vi "Run TCS.vi"(8 "error in (no error)":errorcluster, 11 "SPARC4_GEI in":refnum<class "SPARC4_GEI.lvclass">) -> (0 "error out":errorcluster, 3 "SPARC4_GEI out":refnum<class "SPARC4_GEI.lvclass">)   [LabVIEW 2018, in "SPARC4_GEI.lvclass"]
uses:
  SPARC4_GEI.lvclass
  SPARC4_GEI.lvclass/SPARC4_GEI.ctl
  Filter_Wheel/Filter_Wheel.lvclass/Filter_Wheel.ctl
  State Machine/State Machine.lvclass
  TCS/TCS.lvclass
  Channel GUI/Channel GEI.lvclass
  Filter_Wheel/Filter_Wheel.lvclass
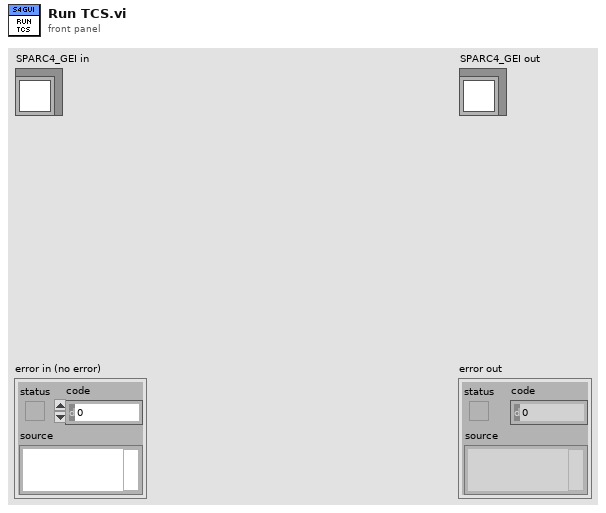
[diagram p1: front panel]
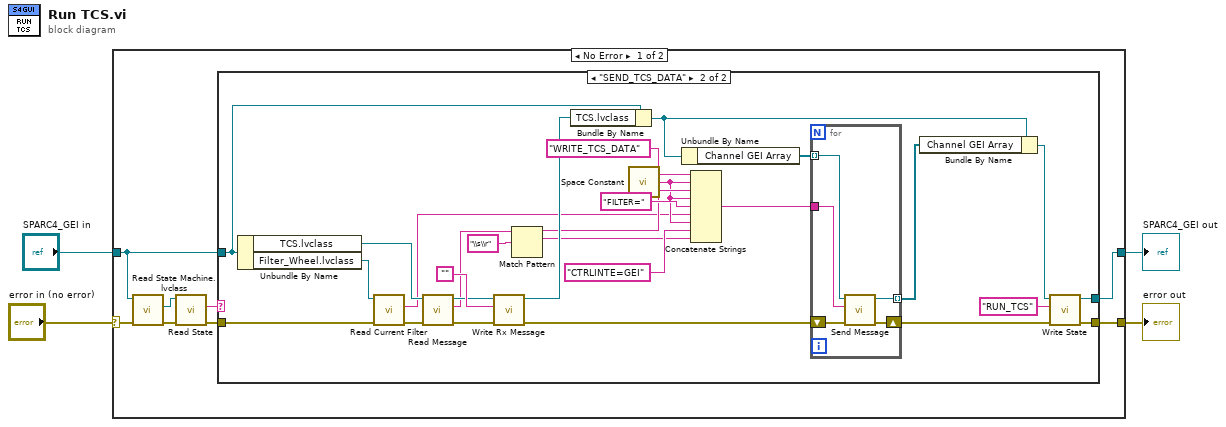
[diagram p0: block diagram]
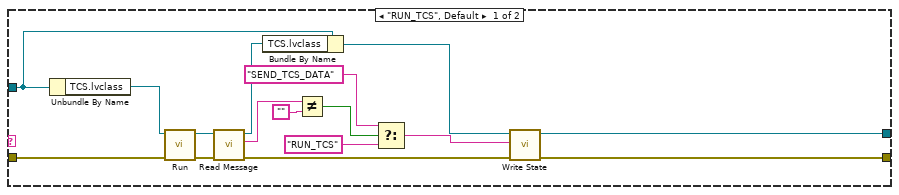
[diagram p2: hidden frame]
diagram:
  n1 = case shown="No Error" "error in (no error)" {
    selector: "error in (no error)" -> [w8 w63]
    tunnel: [w11 w63] -> w3
    tunnel: [w12 w62] -> w2
    tunnel: "SPARC4_GEI in" -> [w5 w62]
    frame No Error {
      n2 = call "Read State Machine.lvclass.vi"("error in (no error)"=w8, "SPARC4_GUI in"=w5) -> ("error out"=w9:errorcluster, "State Machine.lvclass"=w10:refnum<class "State Machine.lvclass">)  [unwired: 7 in, 1 out]
      n3 = call-dynamic "Read State.vi"("error in (no error)"=w9, "State Machine in"=w10) -> ("error out"=w7:errorcluster, "State"=w6:string)  [unwired: 7 in, 1 out]
      n4 = case shown="\"SEND_TCS_DATA\"" w6 {
        tunnel: [w28 w51] -> w12
        tunnel: [w27 w50] -> w11
        tunnel: w7 -> [w15 w31]
        tunnel: w5 -> [w13 w41]
        frame "RUN_TCS", Default {
          n5 = Unbundle By Name(w13) -> ("TCS.lvclass"=w16:refnum<class "TCS.lvclass">)
          n6 = call "Run.vi"("error in (no error)"=w15, "TCS in"=w16) -> ("error out"=w25:errorcluster, "TCS out"=w26:refnum<class "TCS.lvclass">)  [unwired: 8 in]
          n7 = call "Read Message.vi"("error in (no error)"=w25, "TCS in"=w26) -> ("error out"=w23:errorcluster, "Rx Message"=w18:string, "TCS out"=w24:refnum<class "TCS.lvclass">)  [unwired: 7 in]
          n8 = Bundle By Name(cluster=w13, "TCS.lvclass"=w24) -> (w14:refnum<class "SPARC4_GEI.lvclass">)
          n9 = Not Equal?(x=w18, y="") -> (x != y?=w19:bool)
          n10 = Select(t="SEND_TCS_DATA", s=w19, f="RUN_TCS") -> (s? t:f=w22:string)
          n11 = call "Write State.vi"("error in (no error)"=w23, "State"=w22, "SPARC4_GEI in"=w14) -> ("error out"=w27:errorcluster, "SPARC4_GEI out"=w28:refnum<class "SPARC4_GEI.lvclass">)  [unwired: 7 in]
        }
        frame "SEND_TCS_DATA" {
          n12 = Unbundle By Name(w41) -> ("TCS.lvclass"=w42:refnum<class "TCS.lvclass">, "Filter_Wheel.lvclass"=w32:refnum<class "Filter_Wheel.lvclass">)
          n13 = call "Read Current Filter.vi"("error in (no error)"=w31, "Filter_Wheel in"=w32) -> ("error out"=w30:errorcluster, "Current Filter"=w29:string)  [unwired: 7 in, 1 out]
          n14 = call "Read Message.vi"("error in (no error)"=w30, "TCS in"=w42) -> ("error out"=w47:errorcluster, "Rx Message"=w38:string, "TCS out"=w48:refnum<class "TCS.lvclass">)  [unwired: 7 in]
          n15 = call "Write Rx Message.vi"("error in (no error)"=w47, "Rx Message"="", "TCS in"=w48) -> ("error out"=w54:errorcluster, "TCS out"=w53:refnum<class "TCS.lvclass">)  [unwired: 7 in]
          n16 = Match Pattern(string=w38, regular expression="\\s\\r") -> (before substring=w36:string, match substring=w33:string)  [unwired: 1 in, 2 out]
          n17 = Bundle By Name(cluster=w41, "TCS.lvclass"=w53) -> (w55:refnum<class "SPARC4_GEI.lvclass">)
          n18 = call <vilib>:"Space Constant.vi"() -> ("String"=w35:string)
          n19 = Unbundle By Name(w55) -> ("Channel GEI Array"=w56:refnum<class "Channel GEI.lvclass">[])
          n20 = Concatenate Strings("WRITE_TCS_DATA", w35, w36, w35, "FILTER=", w29, w35, "CTRLINTE=GEI", w33) -> (w44:string)
          n21 = for {
            tunnel: w44 -> [w58]
            tunnel: w56 -> [w57] mode=indexing
            tunnel: [w61] -> w46 mode=indexing
            shift-right: [w60] -> w45
            shift-left: w54 -> [w59]
            n22 = call "Send Message.vi"("error in (no error)"=w59, "Message"=w58, "Channel GUI in"=w57) -> ("error out"=w60:errorcluster, "Channel GUI out"=w61:refnum<class "Channel GEI.lvclass">)  [unwired: 7 in]
          }
          n23 = Bundle By Name(cluster=w55, "Channel GEI Array"=w46) -> (w40:refnum<class "SPARC4_GEI.lvclass">)
          n24 = call "Write State.vi"("error in (no error)"=w45, "State"="RUN_TCS", "SPARC4_GEI in"=w40) -> ("error out"=w50:errorcluster, "SPARC4_GEI out"=w51:refnum<class "SPARC4_GEI.lvclass">)  [unwired: 7 in]
        }
      }
    }
    frame Error {
    }
  }
  "error out" <- w3
  "SPARC4_GEI out" <- w2
